vi "ReceiveData.vi"(8 "error in (no error)":errorcluster, 10 "Def-ReceiveData":T1={"Channel Num"=0, "timeout(ms)"=50}, 11 "CAN-NI in":refnum<class "CAN-NI.lvclass">) -> (0 "error out":errorcluster, 2 "FrameData":T2, 3 "CAN-NI out":refnum<class "CAN-NI.lvclass">)   [LabVIEW 2019, in "CAN-NI.lvlib" / "CAN-NI.lvclass"]
uses:
  CAN-NI.lvclass
  CAN-Interface/TypeDef/Def-CANData.ctl
  CAN-Interface/TypeDef/Def-ReceiveData.ctl
  <vilib>/xnet/xnet.llb/XNET Read (Frame CAN).vi
  CAN-Interface/Class-Interface.lvclass
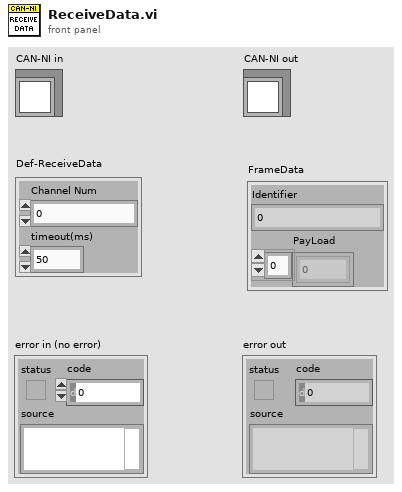
[diagram p1: front panel]
types:
  T1 = typedef "CAN-Interface.lvlib/Class-Interface.lvclass/Def-ReceiveData.ctl" = cluster{"Channel Num":u32, "timeout(ms)":i32}
  T2 = typedef "CAN-Interface.lvlib/Class-Interface.lvclass/Def-CANData.ctl" = cluster{"Identifier":u32, "PayLoad":u8[]}
  T3 = typedef "CAN-NI.lvlib/CAN-NI.lvclass/ChannelProperty.ctl" = cluster{"CAN-cluster":refnum<k21>, "CAN-Frames":refnum<k21>[], "Termination":T4, "Transmit Mode":T5, "Frame Out Session":refnum<k21>, "Frame In Session":refnum<k21>, "Protocol":T6}
  T4 = typedef "CAN-Interface.lvlib/Class-Interface.lvclass/Def-Termination.ctl" = enum8{"on", "off"}
  T5 = typedef "CAN-Interface.lvlib/Class-Interface.lvclass/Def-Transmit Mode.ctl" = enum16{"Queued", "Stream"}
  T6 = typedef "CAN-Interface.lvlib/Class-Interface.lvclass/Def-Protocol.ctl" = enum16{"CAN", "CAN FD"}
  T7 = typedef "XNET Frame CAN.ctl" = cluster{"timestamp":timestamp, "payload":u8[], "identifier":u32, "type":T8, "extended?":bool, "echo?":bool}
  T8 = typedef "XNET Frame Type CAN.ctl" = u8
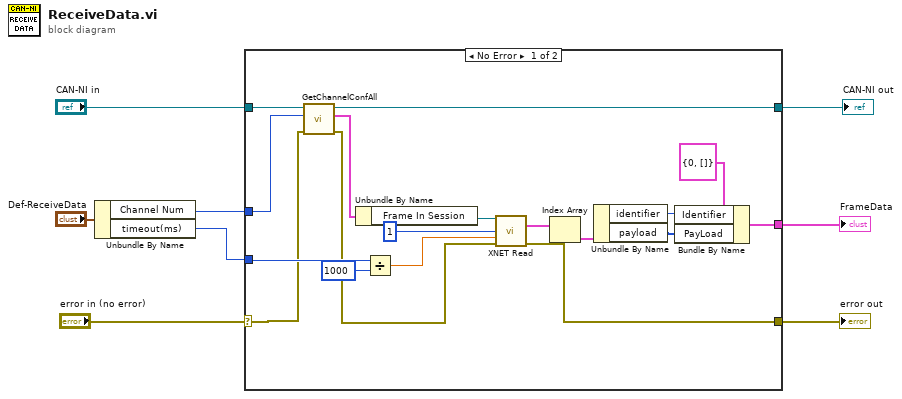
[diagram p0: block diagram]
diagram:
  n1 = Unbundle By Name("Def-ReceiveData") -> ("Channel Num"=w3:u32, "timeout(ms)"=w2:i32)
  n2 = case shown="No Error" "error in (no error)" {
    selector: "error in (no error)" -> [w11 w28]
    tunnel: "CAN-NI in" -> [w26 w27]
    tunnel: w3 -> [w25 _]
    tunnel: [w22 _] -> w1
    tunnel: [w21 w28] -> w6
    tunnel: [w20 w27] -> w5
    tunnel: w2 -> [w19 _]
    frame No Error {
      n3 = call "GetChannelConfAll.vi"("error in"=w11, "Channel Num"=w25, "CAN-NI"=w26) -> ("error out"=w9:errorcluster, "ChannelProperty"=w24:T3, "CAN-NI"=w20:refnum<class "CAN-NI.lvclass">)  [unwired: 6 in]
      n4 = Unbundle By Name(w24) -> ("Frame In Session"=w23:refnum<k21>)
      n5 = Divide(x=w19, y=1000) -> (x/y=w17:dbl)
      n6 = call-poly <vilib>:"XNET Read.vi"("session in"=w23, "number to read (-1)"=1, "timeout (0)"=w17, "error in (no error)"=w9) -> ("data"=w13:T7[], "error out"=w21:errorcluster)  [unwired: 8 in, 2 out]
      n7 = Index Array(array=w13) -> (element=w12:T7)  [unwired: 1 in]
      n8 = Unbundle By Name(w12) -> ("identifier"=w16:u32, "payload"=w14:u8[])
      n9 = Bundle By Name(cluster=T2 {"Identifier"=0, "PayLoad"=[]} ("CANData"), "Identifier"=w16, "PayLoad"=w14) -> (w22:T2)
    }
    frame Error {
    }
  }
  "error out" <- w6
  "CAN-NI out" <- w5
  "FrameData" <- w1
